vi "Enqueue CTRL Element.vi"(8 "error in (no error)":errorcluster, 10 "Control Data":T1, 11 "CTRL Data Queue in":refnum<queue>) -> (0 "error out":errorcluster, 3 "CTRL Data Queue out":refnum<queue>)   [LabVIEW 2014, in "WINFAS 2 Data Queue.lvlib"]
uses:
  WINFAS 2 Data Queue.lvlib
  Control Data Cluster.ctl
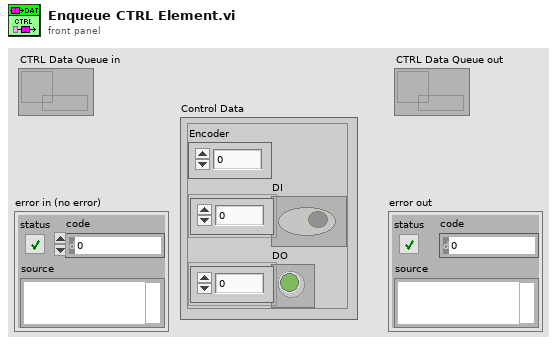
[diagram p1: front panel]
types:
  T1 = typedef "WINFAS 2 Data Queue.lvlib/Control Data Cluster.ctl" = cluster{"Encoder":sgl, "DI":bool[], "DO":bool[]}
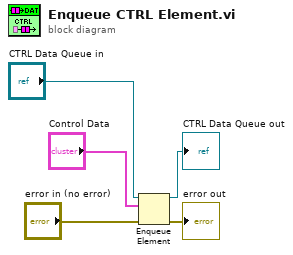
[diagram p0: block diagram]
diagram:
  n1 = Enqueue Element(queue="CTRL Data Queue in", element="Control Data", error in (no error)="error in (no error)") -> (queue out=→"CTRL Data Queue out":refnum<queue>, error out=→"error out":errorcluster)  [unwired: 1 in, 1 out]
